vi "Wrt_TimeTable.vi"(7 "ReadOnlyIn":T11={"Qref"={"ValveCTR"=refnum, "Error"=refnum}, "UI_EN"=FALSE, "UserEventREF"={"TimeBasedProducer"={"Reg"=refnum, "Ref"=refnum}, "TimeBasedTempRead"={"Reg"=refnum, "Ref"=refnum}}, "UI_REF"=variant(cluster{} {}), "Paths"={"Log_Dir"=path "", "TempLog"=path "", "WateringLog"=path "", "Error"=path "", "Settings_Dir"=path "", "CFG.ini"=path "", "Plant_Digital_OP"=path "", "TimeTable"=path "", "Consol_Dir"=path "", "Input"=path "", "Output"=path "", "Timeout"=path "", "TimeoutTable"=path "", "Ch_Stat"=path "", "Temp"=path ""}, "PI_REF"={"IO"=enum."Remote", "Interface"=enum."Serial", "LINX Device Config"={"Interface"=enum."Serial", "COM Port"="COM13", "TCP Configuration"={"IP Address"="", "Port"=0}, "Device Family"=1, "Device ID"=1, "Device Name"="myRIO-1900", "TCP Ref"=refnum, "Channels"={"DI"=[0, 1, 2, 3, 4, 5, 6, 7, 8, 9, 10, 11, 12, 13, 14, 15, 16, 17, 18, 19, 20, 21, 22, 23, 24, 25, 26, 27, 28, 29, 30, 31, 32, 33, 34, 35, 36, 37, 38, 39, 40, 41, 42, 43, 44, 45, 46], "DO"=[0, 1, 2, 3, 4, 5, 6, 7, 8, 9, 10, 11, 12, 13, 14, 15, 16, 17, 18, 19, 20, 21, 22, 23, 24, 25, 26, 27, 28, 29, 30, 31, 32, 33, 34, 35, 36, 37, 38, 39, 40, 41, 42, 43, 44, 45, 46], "AI"=[0, 1, 2, 3, 4, 5, 6, 7, 8, 9, 10, 11], "AO"=[], "PWM"=[3, 5, 6, 9, 10], "QE"=[], "UART"=[0, 1], "I2C 2"=[0], "SPI"=[0], "CAN"=[], "Servo"=[], "AI Ref (V)"=0.0, "AI Resolution (Bits)"=0, "AO Ref (V)"=0.0, "AO Resolution (Bits)"=0}}}, "CFG"={"ProducerEn_PC"=FALSE, "Producer_PC_ms"=0, "ProducerEn_PI"=FALSE, "Producer_PI_ms"=0, "TempLogInterval"=15, "SystemResetTime"=0.0}} {"CFG"."SystemResetTime" format="%<%H:%M:%S>t"}, 8 "Error In":errorcluster, 9 "Time Table In":T2=[{"Set Time"=0.0, "Control"=enum."Time", "Duration[S]"=3.0, "Liter"=0.0, "Plant Name."="", "Watered"=FALSE, "Su"=FALSE, "Mo"=FALSE, "Tu"=FALSE, "We"=FALSE, "Th"=FALSE, "Fr"=FALSE, "Sa"=FALSE}, {"Set Time"=0.0, "Control"=enum."Time", "Duration[S]"=5.0, "Liter"=0.0, "Plant Name."="", "Watered"=FALSE, "Su"=FALSE, "Mo"=FALSE, "Tu"=FALSE, "We"=FALSE, "Th"=FALSE, "Fr"=FALSE, "Sa"=FALSE}, {"Set Time"=0.0, "Control"=enum."Time", "Duration[S]"=5.0, "Liter"=0.0, "Plant Name."="", "Watered"=FALSE, "Su"=FALSE, "Mo"=FALSE, "Tu"=FALSE, "We"=FALSE, "Th"=FALSE, "Fr"=FALSE, "Sa"=FALSE}] {"Liter" min=0.0; "Set Time" format="%<%H:%M:%S>t"; "Duration[S]" min=0.0}, 10 "RST_Flag":bool, 11 "Read_WriteIN":T1={"Time Table"=[{"Set Time"=0.0, "Control"=enum."Time", "Duration[S]"=3.0, "Liter"=0.0, "Plant Name."="", "Watered"=FALSE, "Su"=FALSE, "Mo"=FALSE, "Tu"=FALSE, "We"=FALSE, "Th"=FALSE, "Fr"=FALSE, "Sa"=FALSE}, {"Set Time"=0.0, "Control"=enum."Time", "Duration[S]"=5.0, "Liter"=0.0, "Plant Name."="", "Watered"=FALSE, "Su"=FALSE, "Mo"=FALSE, "Tu"=FALSE, "We"=FALSE, "Th"=FALSE, "Fr"=FALSE, "Sa"=FALSE}, {"Set Time"=0.0, "Control"=enum."Time", "Duration[S]"=5.0, "Liter"=0.0, "Plant Name."="", "Watered"=FALSE, "Su"=FALSE, "Mo"=FALSE, "Tu"=FALSE, "We"=FALSE, "Th"=FALSE, "Fr"=FALSE, "Sa"=FALSE}], "Plants_Digital_OP"=[], "delta_ms_w_Index"={"delta_ms"=[], "Index"=[], "RunArray"=[]}, "TimeOutInfo"={"Timeout"=0, "ValveCTR"={"State"=enum."Open Valve", "Channel No"=0, "Duration[S]"=0.0}, "Index"=0}, "LoopName"=""} {"TimeOutInfo"."ValveCTR"."Channel No" items=["7"=7, "11"=11, "12"=12, "13"=13, "15"=15, "16"=16, "18"=18, "29"=29, "32"=32, "33"=33, "35"=35, "36"=36, "37"=37, "38"=38, "40"=40]; "delta_ms_w_Index"."RunArray"."Channel No" items=["7"=7, "11"=11, "12"=12, "13"=13, "15"=15, "16"=16, "18"=18, "29"=29, "32"=32, "33"=33, "35"=35, "36"=36, "37"=37, "38"=38, "40"=40]; "Plants_Digital_OP"."Channel No" items=["7"=7, "11"=11, "12"=12, "13"=13, "15"=15, "16"=16, "18"=18, "29"=29, "32"=32, "33"=33, "35"=35, "36"=36, "37"=37, "38"=38, "40"=40]; "Time Table"."Liter" min=0.0; "Time Table"."Set Time" format="%<%H:%M:%S>t"; "Time Table"."Duration[S]" min=0.0}) -> (0 "Error Out":errorcluster, 3 "Read_WriteOUT":T1={"Time Table"=[{"Set Time"=0.0, "Control"=enum."Time", "Duration[S]"=3.0, "Liter"=0.0, "Plant Name."="", "Watered"=FALSE, "Su"=FALSE, "Mo"=FALSE, "Tu"=FALSE, "We"=FALSE, "Th"=FALSE, "Fr"=FALSE, "Sa"=FALSE}, {"Set Time"=0.0, "Control"=enum."Time", "Duration[S]"=5.0, "Liter"=0.0, "Plant Name."="", "Watered"=FALSE, "Su"=FALSE, "Mo"=FALSE, "Tu"=FALSE, "We"=FALSE, "Th"=FALSE, "Fr"=FALSE, "Sa"=FALSE}, {"Set Time"=0.0, "Control"=enum."Time", "Duration[S]"=5.0, "Liter"=0.0, "Plant Name."="", "Watered"=FALSE, "Su"=FALSE, "Mo"=FALSE, "Tu"=FALSE, "We"=FALSE, "Th"=FALSE, "Fr"=FALSE, "Sa"=FALSE}], "Plants_Digital_OP"=[], "delta_ms_w_Index"={"delta_ms"=[], "Index"=[], "RunArray"=[]}, "TimeOutInfo"={"Timeout"=0, "ValveCTR"={"State"=enum."Open Valve", "Channel No"=0, "Duration[S]"=0.0}, "Index"=0}, "LoopName"=""} {"TimeOutInfo"."ValveCTR"."Channel No" items=["7"=7, "11"=11, "12"=12, "13"=13, "15"=15, "16"=16, "18"=18, "29"=29, "32"=32, "33"=33, "35"=35, "36"=36, "37"=37, "38"=38, "40"=40]; "delta_ms_w_Index"."RunArray"."Channel No" items=["7"=7, "11"=11, "12"=12, "13"=13, "15"=15, "16"=16, "18"=18, "29"=29, "32"=32, "33"=33, "35"=35, "36"=36, "37"=37, "38"=38, "40"=40]; "Plants_Digital_OP"."Channel No" items=["7"=7, "11"=11, "12"=12, "13"=13, "15"=15, "16"=16, "18"=18, "29"=29, "32"=32, "33"=33, "35"=35, "36"=36, "37"=37, "38"=38, "40"=40]; "Time Table"."Liter" min=0.0; "Time Table"."Set Time" format="%<%H:%M:%S>t"; "Time Table"."Duration[S]" min=0.0})   [LabVIEW 2014, in "TimeBasedProd.lvlib"]
uses:
  TimeBasedProd.lvlib
  TypeDef/Time_Table.ctl
  TypeDef/Time_Table_CTR.ctl
  Main/TypeDef/ReadOnly.ctl
  ValveCTRL/TypeDef/Queue_Cluster.ctl
  ValveCTRL/TypeDef/States_Enum.ctl
  ValveCTRL/TypeDef/CHs_List.ctl
  Main/TypeDef/EventData.ctl
  <vilib>/MakerHub/LINX/Private/Type Defs/LINX Ref.ctl
  <vilib>/MakerHub/LINX/Private/Type Defs/Platform.ctl
  <vilib>/MakerHub/LINX/Private/Type Defs/Interface.ctl
  <vilib>/MakerHub/LINX/Private/Device/Type Defs/LINX Device Config.ctl
  <vilib>/MakerHub/LINX/Private/Device/Type Defs/TCP Config.ctl
  <vilib>/MakerHub/LINX/Private/Device/Type Defs/Channels.ctl
  Main/Init/ReadInitCFG/TypeDef/CFG_Cluster.ctl
  TypeDef/Read_Write.ctl
  Digital_OP/TypeDef/Plant_OP_Map.ctl
  Digital_OP/TypeDef/Plant_OP_Map_CTR.ctl
  TypeDef/TimeOutInfo.ctl
  TypeDef/UpdateTimeOutinfo.ctl
  <vilib>/Utility/file.llb/Write To Spreadsheet File (string).vi
  ValveCTRL/ValveCTRL.lvlib
  Main/Main.lvlib
  <vilib>/MakerHub/LINX/LMH-LINX.lvlib
  <vilib>/MakerHub/LINX/Private/Device/Device.lvlib
panel:
  # "Watering Days"
  # "Watering Days"
  # "Watering Days"
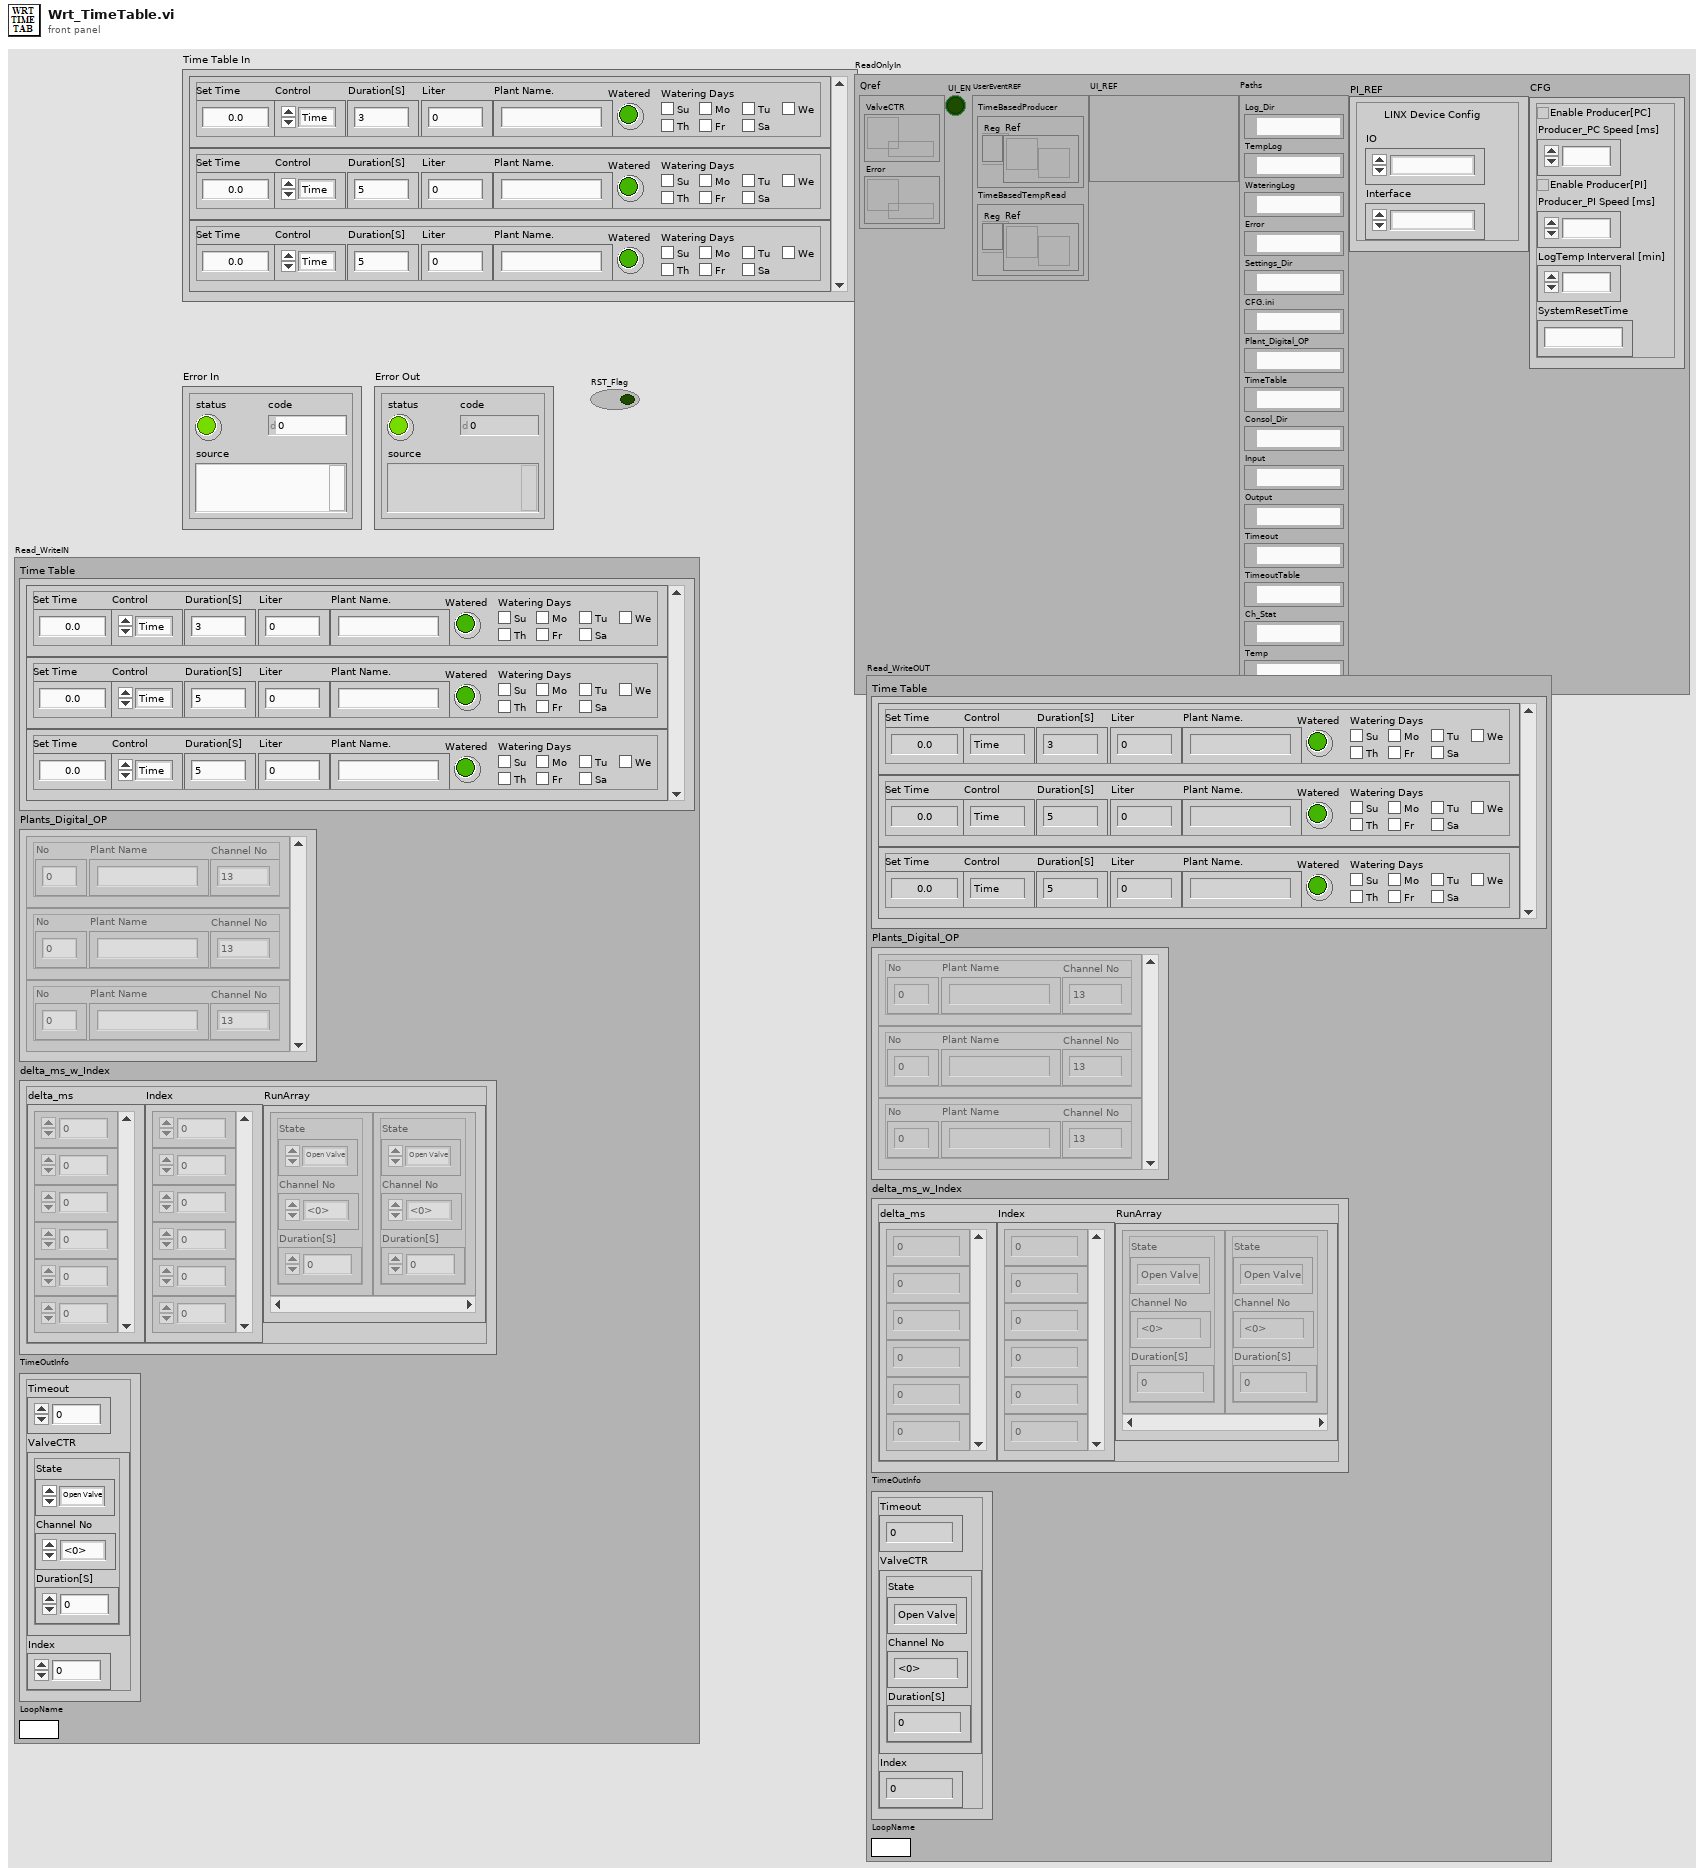
[diagram p1: front panel]
types:
  T1 = typedef "TimeBasedProd.lvlib/Read_Write.ctl" = cluster{"Time Table":T2, "Plants_Digital_OP":T4, "delta_ms_w_Index":T7, "TimeOutInfo":T10, "LoopName":string}
  T2 = typedef "TimeBasedProd.lvlib/Time_Table.ctl" = T3[]
  T3 = typedef "TimeBasedProd.lvlib/Time_Table_CTR.ctl" = cluster{"Set Time":dbl, "Control":enum16{"Time", "Flow"}, "Duration[S]":dbl, "Liter":dbl, "Plant Name.":string, "Watered":bool, "Su":bool, "Mo":bool, "Tu":bool, "We":bool, "Th":bool, "Fr":bool, "Sa":bool}
  T4 = typedef "TimeBasedProd.lvlib/Plant_OP_Map.ctl" = T5[]
  T5 = typedef "TimeBasedProd.lvlib/Plant_OP_Map_CTR.ctl" = cluster{"No":u8, "Plant Name":string, "Channel No":T6}
  T6 = typedef "ValveCTRL.lvlib/CHs_List.ctl" = u8
  T7 = typedef "TimeBasedProd.lvlib/TimeOutInfo.ctl" = cluster{"delta_ms":i32[], "Index":i32[], "RunArray":T8[]}
  T8 = typedef "ValveCTRL.lvlib/Queue_Cluster.ctl" = cluster{"State":T9, "Channel No":T6, "Duration[S]":dbl}
  T9 = typedef "ValveCTRL.lvlib/States_Enum.ctl" = enum16{"Open Pump", "Open Valve", "Wait Valve", "Close Pump", "Close Valve", "Save State", "StopLoop", "ValidCh"}
  T10 = typedef "TimeBasedProd.lvlib/UpdateTimeOutinfo.ctl" = cluster{"Timeout":i32, "ValveCTR":T8, "Index":i32}
  T11 = typedef "Main.lvlib/ReadOnly.ctl" = cluster{"Qref":cluster{"ValveCTR":refnum<queue>, "Error":refnum<queue>}, "UI_EN":bool, "UserEventREF":cluster{"TimeBasedProducer":cluster{"Reg":refnum<event-registration>, "Ref":refnum<user-event>}, "TimeBasedTempRead":cluster{"Reg":refnum<event-registration>, "Ref":refnum<user-event>}}, "UI_REF":variant, "Paths":cluster{"Log_Dir":path, "TempLog":path, "WateringLog":path, "Error":path, "Settings_Dir":path, "CFG.ini":path, "Plant_Digital_OP":path, "TimeTable":path, "Consol_Dir":path, "Input":path, "Output":path, "Timeout":path, "TimeoutTable":path, "Ch_Stat":path, "Temp":path}, "PI_REF":T12, "CFG":T18}
  T12 = typedef "LMH-LINX.lvlib/LINX Ref.ctl" = cluster{"IO":T13, "Interface":T14, "LINX Device Config":T15}
  T13 = typedef "LMH-LINX.lvlib/Platform.ctl" = enum16{"Remote", "Local"}
  T14 = typedef "LMH-LINX.lvlib/Interface.ctl" = enum16{"Serial", "TCP"}
  T15 = typedef "LMH-LINX.lvlib/Device.lvlib/LINX Device Config.ctl" = cluster{"Interface":T14, "COM Port":refnum<visa-resource-name>, "TCP Configuration":T16, "Device Family":u8, "Device ID":u8, "Device Name":string, "TCP Ref":refnum<k5>, "Channels":T17}
  T16 = typedef "LMH-LINX.lvlib/Device.lvlib/TCP Config.ctl" = cluster{"IP Address":string, "Port":u16}
  T17 = typedef "LMH-LINX.lvlib/Channels.ctl" = cluster{"DI":u8[], "DO":u8[], "AI":u8[], "AO":u8[], "PWM":u8[], "QE":u8[], "UART":u8[], "I2C 2":u8[], "SPI":u8[], "CAN":u8[], "Servo":u8[], "AI Ref (V)":dbl, "AI Resolution (Bits)":u8, "AO Ref (V)":dbl, "AO Resolution (Bits)":u8}
  T18 = typedef "Main.lvlib/CFG_Cluster.ctl" = cluster{"ProducerEn_PC":bool, "Producer_PC_ms":u32, "ProducerEn_PI":bool, "Producer_PI_ms":u32, "TempLogInterval":u32, "SystemResetTime":dbl}
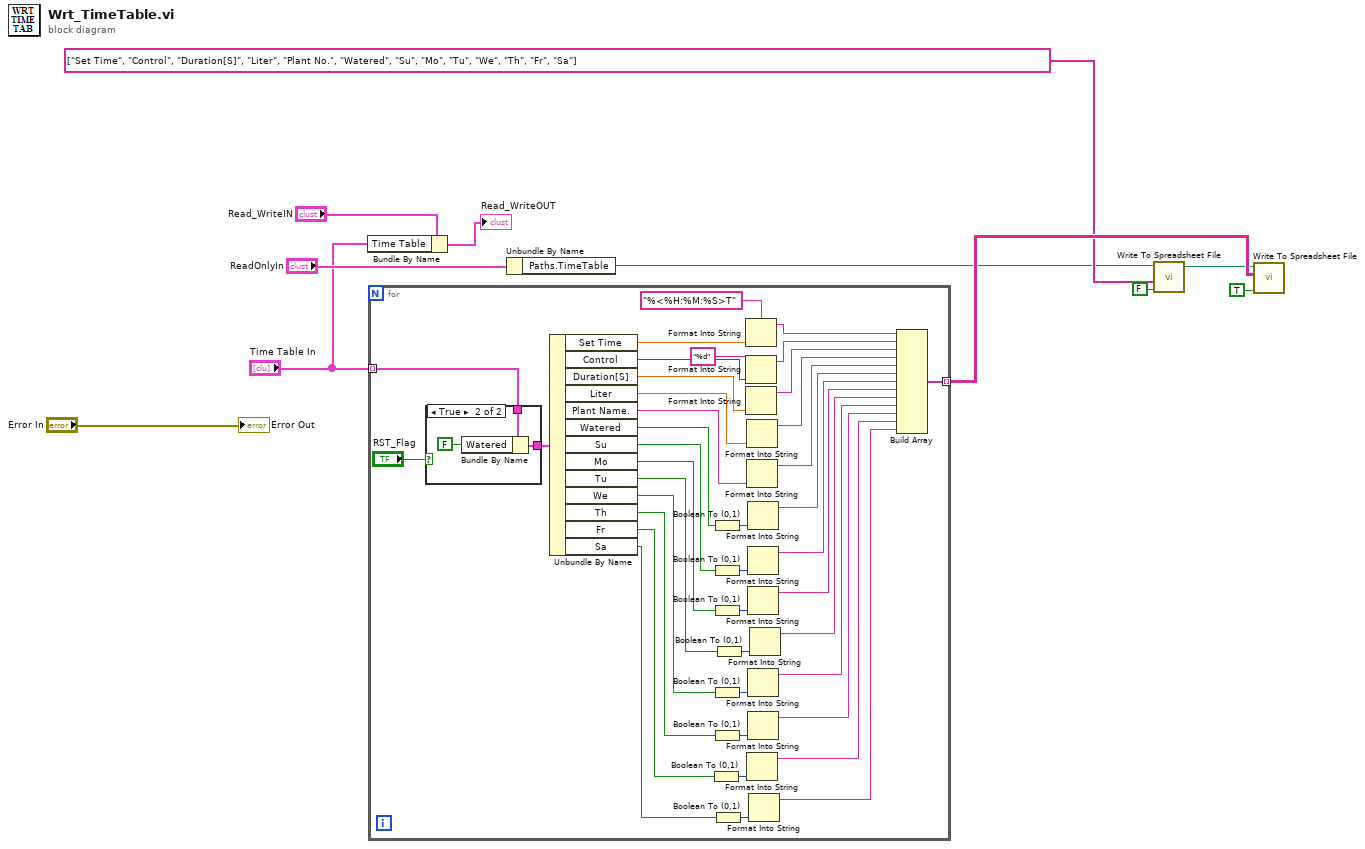
[diagram p0: block diagram]
diagram:
  n1 = Bundle By Name(cluster="Read_WriteIN", "Time Table"="Time Table In") -> (→"Read_WriteOUT":T1)
  n2 = for {
    tunnel: "Time Table In" -> [w15] mode=indexing
    tunnel: [w48] -> w11 mode=indexing
    n3 = case shown="True" "RST_Flag" {
      tunnel: w15 -> [w52 w55]
      tunnel: [w52 w54] -> w14
      frame False {
      }
      frame True {
        n4 = Bundle By Name(cluster=w55, "Watered"=FALSE) -> (w54:T3)
      }
    }
    n5 = Unbundle By Name(w14) -> ("Set Time"=w12:dbl, "Control"=w49:enum16{"Time", "Flow"}, "Duration[S]"=w46:dbl, "Liter"=w45:dbl, "Plant Name."=w40:string, "Watered"=w38:bool, "Su"=w32:bool, "Mo"=w31:bool, "Tu"=w30:bool, "We"=w29:bool, "Th"=w23:bool, "Fr"=w19:bool, "Sa"=w16:bool)
    n6 = Boolean To (0,1)(Boolean=w19) -> (0, 1=w21:i16)
    n7 = Boolean To (0,1)(Boolean=w38) -> (0, 1=w37:i16)
    n8 = Boolean To (0,1)(Boolean=w32) -> (0, 1=w36:i16)
    n9 = Boolean To (0,1)(Boolean=w31) -> (0, 1=w35:i16)
    n10 = Boolean To (0,1)(Boolean=w29) -> (0, 1=w33:i16)
    n11 = Boolean To (0,1)(Boolean=w23) -> (0, 1=w24:i16)
    n12 = Boolean To (0,1)(Boolean=w16) -> (0, 1=w18:i16)
    n13 = Boolean To (0,1)(Boolean=w30) -> (0, 1=w34:i16)
    n14 = Format Into String(format string="%<%H:%M:%S>T", w12) -> (resulting string=w51:string)  [unwired: 2 in, 1 out]
    n15 = Format Into String(format string="%d", w49) -> (resulting string=w50:string)  [unwired: 2 in, 1 out]
    n16 = Format Into String(w46) -> (resulting string=w47:string)  [unwired: 3 in, 1 out]
    n17 = Format Into String(w45) -> (resulting string=w44:string)  [unwired: 3 in, 1 out]
    n18 = Format Into String(w40) -> (resulting string=w41:string)  [unwired: 3 in, 1 out]
    n19 = Format Into String(w21) -> (resulting string=w20:string)  [unwired: 3 in, 1 out]
    n20 = Format Into String(w37) -> (resulting string=w39:string)  [unwired: 3 in, 1 out]
    n21 = Format Into String(w36) -> (resulting string=w28:string)  [unwired: 3 in, 1 out]
    n22 = Format Into String(w35) -> (resulting string=w27:string)  [unwired: 3 in, 1 out]
    n23 = Format Into String(w33) -> (resulting string=w25:string)  [unwired: 3 in, 1 out]
    n24 = Format Into String(w24) -> (resulting string=w22:string)  [unwired: 3 in, 1 out]
    n25 = Format Into String(w18) -> (resulting string=w17:string)  [unwired: 3 in, 1 out]
    n26 = Format Into String(w34) -> (resulting string=w26:string)  [unwired: 3 in, 1 out]
    n27 = Build Array(w51, w50, w47, w44, w41, w39, w28, w27, w26, w25, w22, w20, w17) -> (w48:string[])
  }
  n28 = Unbundle By Name("ReadOnlyIn") -> ("Paths.TimeTable"=w4:path)
  n29 = call-poly <vilib>:"Write To Spreadsheet File.vi"("append to file? (new file:F)"=FALSE, "1D data"=string[] ["Set Time", "Control", "Duration[S]", "Liter", "Plant No.", "Watered", "Su", "Mo", "Tu", "We", "Th", "Fr", "Sa"], "file path (dialog if empty)"=w4) -> ("new file path (Not A Path if cancelled)"=w9:path)  [unwired: 5 in]
  n30 = call-poly <vilib>:"Write To Spreadsheet File.vi"("append to file? (new file:F)"=TRUE, "2D data"=w11, "file path (dialog if empty)"=w9) -> ()  [unwired: 5 in, 1 out]
  "Error Out" <- "Error In"
